vi "filter.debug.vi"(11 "filter.data in":T1 {"memory.command"."order.slot.value"."Quantity" format="%016x"; "memory.command"."order.slot.value"."OrderId" format="%016x"; "memory.command"."ticker.slot.value"."Symbol" format="%016x"; "Scratch"."OrderId" format="%016x"}) -> (3 "filter.data out":T1 {"memory.command"."order.slot.value"."Quantity" format="%016x"; "memory.command"."order.slot.value"."OrderId" format="%016x"; "memory.command"."ticker.slot.value"."Symbol" format="%016x"; "Scratch"."OrderId" format="%016x"})   [LabVIEW 2022 SP3]
uses:
  filter.data.ctl
  filter.states.ctl
  filter.debug.ctl
  filter.debug.slot.ctl
  filter.data.scratch.ctl
  common/orderbook.command.ctl
  common/orderbook.command.type.ctl
  filter.memory.command.ctl
  ticker.slot.ctl
  order.slot.ctl
  filter.getstate.ctl
  filter.getstate.slot.ctl
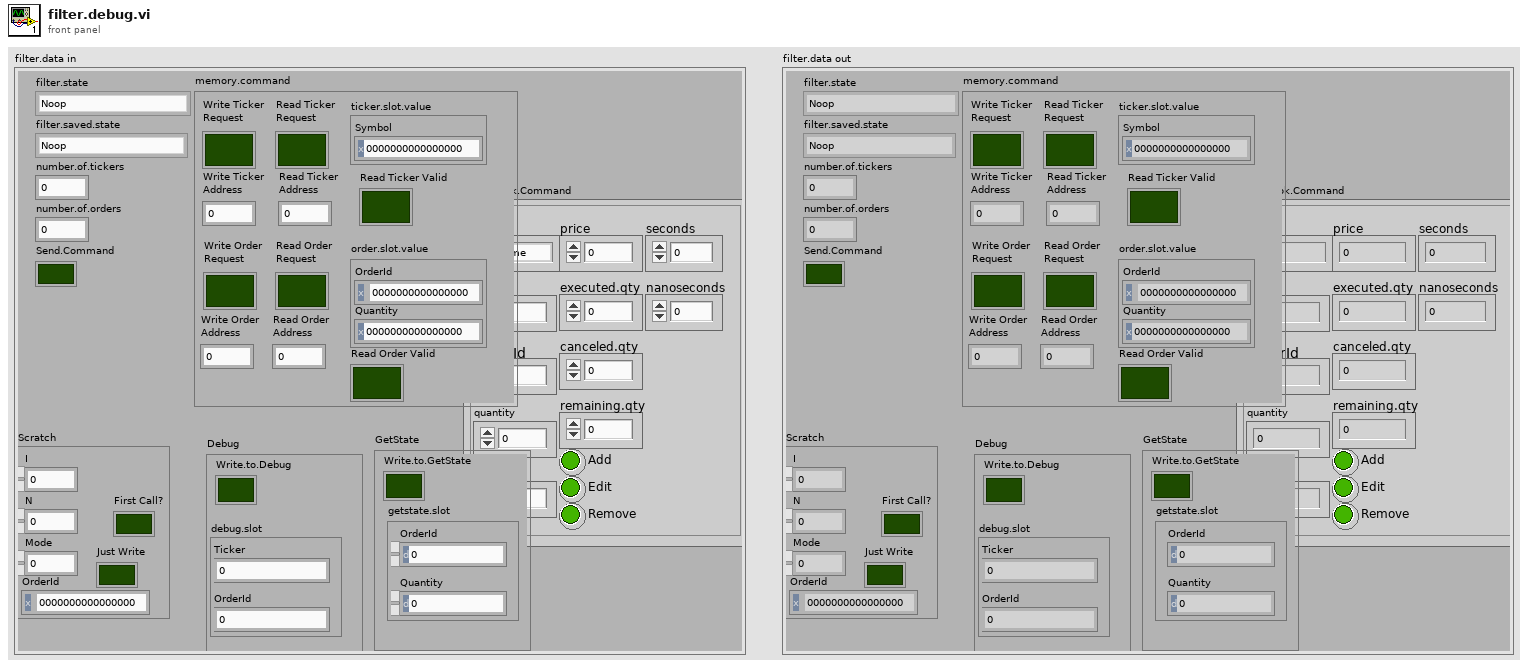
[diagram p1: front panel]
types:
  T1 = typedef "filter.data.ctl" = cluster{"filter.state":T2, "Debug":T3, "number.of.tickers":u32, "number.of.orders":u32, "filter.saved.state":T2, "Scratch":T5, "OrderBook.Command":T6, "Send.Command":bool, "memory.command":T8, "GetState":T11}
  T2 = typedef "filter.states.ctl" = enum16{"Noop", "Reset", "Debug", "Configuration", "Get.State", "Wait.for.Command", "Filter.Add", "Filter.Other", "Insert.Order", "Delete Order"}
  T3 = typedef "filter.debug.ctl" = cluster{"Write.to.Debug":bool, "debug.slot":T4}
  T4 = typedef "filter.debug.slot.ctl" = cluster{"Ticker":u64, "OrderId":u64}
  T5 = typedef "filter.data.scratch.ctl" = cluster{"I":u32, "N":u32, "Mode":u32, "OrderId":u64, "First Call?":bool, "Just Write":bool}
  T6 = typedef "orderbook.command.ctl" = cluster{"type":T7, "side":u8, "orderId ":u64, "quantity":u32, "symbol":u64, "price":u64, "executed.qty":u32, "canceled.qty":u32, "remaining.qty":u32, "seconds":u64, "nanoseconds":u64, "Add":bool, "Edit":bool, "Remove":bool}
  T7 = typedef "orderbook.command.type.ctl" = enum8{"Time", "AddOrder", "OrderExecuted", "OrderExecutedAtPrice", "ReduceSize", "ModifyOrder", "DeleteOrder", "Get.Everything", "Get.All.Orders", "Get.Top"}
  T8 = typedef "filter.memory.command.ctl" = cluster{"ticker.slot.value":T9, "order.slot.value":T10, "Write Ticker\nAddress":u32, "Write Ticker\nRequest":bool, "Read Ticker\nRequest":bool, "Read Ticker\nAddress":u32, "Read Ticker Valid":bool, "Write Order\nAddress":u32, "Write Order\nRequest":bool, "Read Order\nRequest":bool, "Read Order\nAddress":u32, "Read Order Valid":bool}
  T9 = typedef "ticker.slot.ctl" = cluster{"Symbol":u64}
  T10 = typedef "order.slot.ctl" = cluster{"OrderId":u64, "Quantity":u64}
  T11 = typedef "filter.getstate.ctl" = cluster{"Write.to.GetState":bool, "getstate.slot":T12}
  T12 = typedef "filter.getstate.slot.ctl" = cluster{"OrderId":u64, "Quantity":u64}
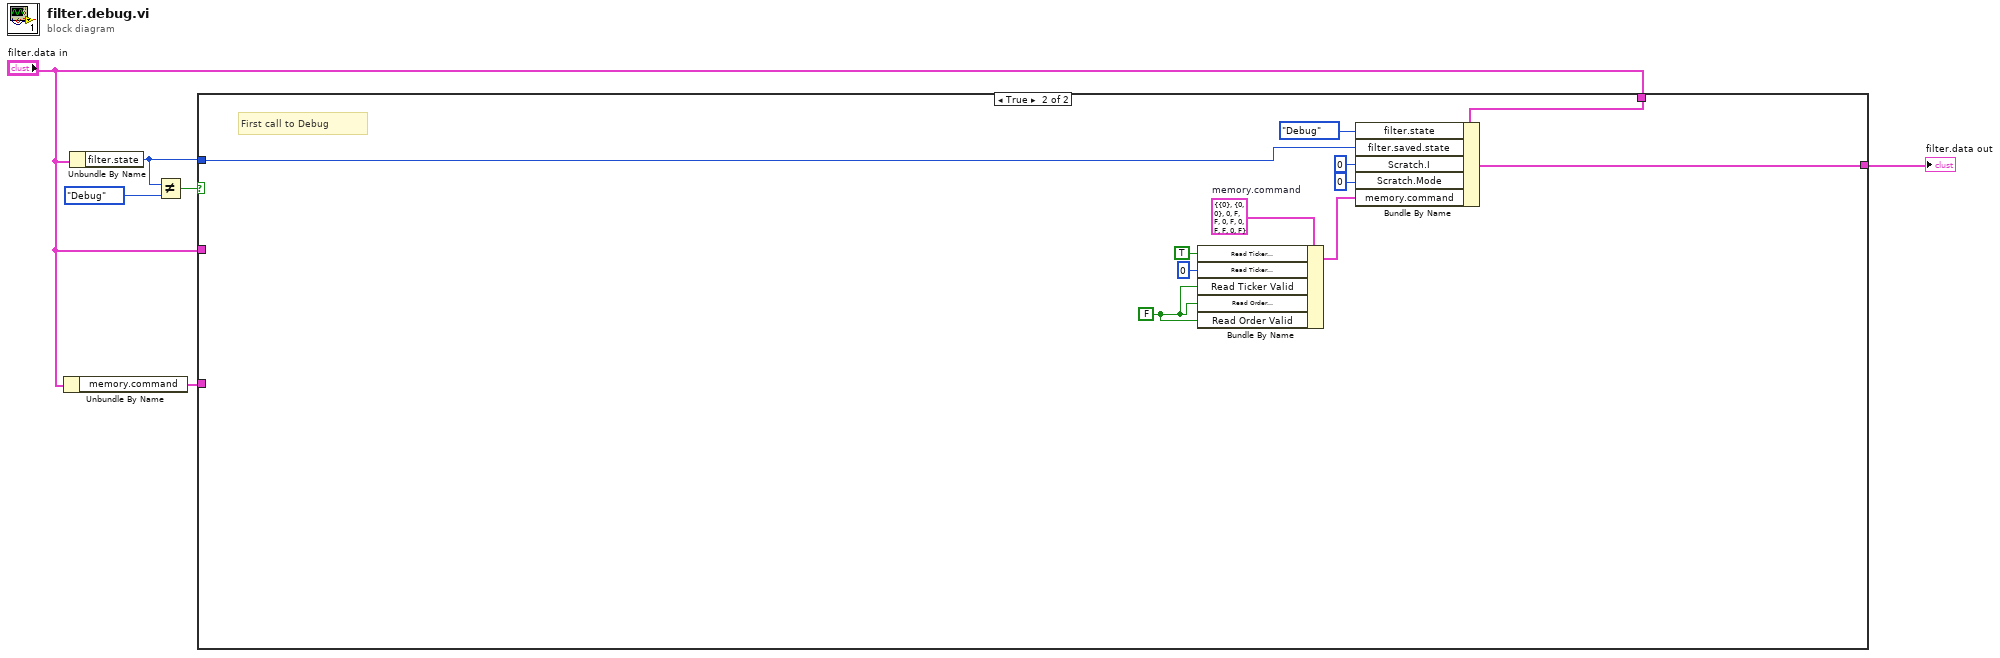
[diagram p0: block diagram]
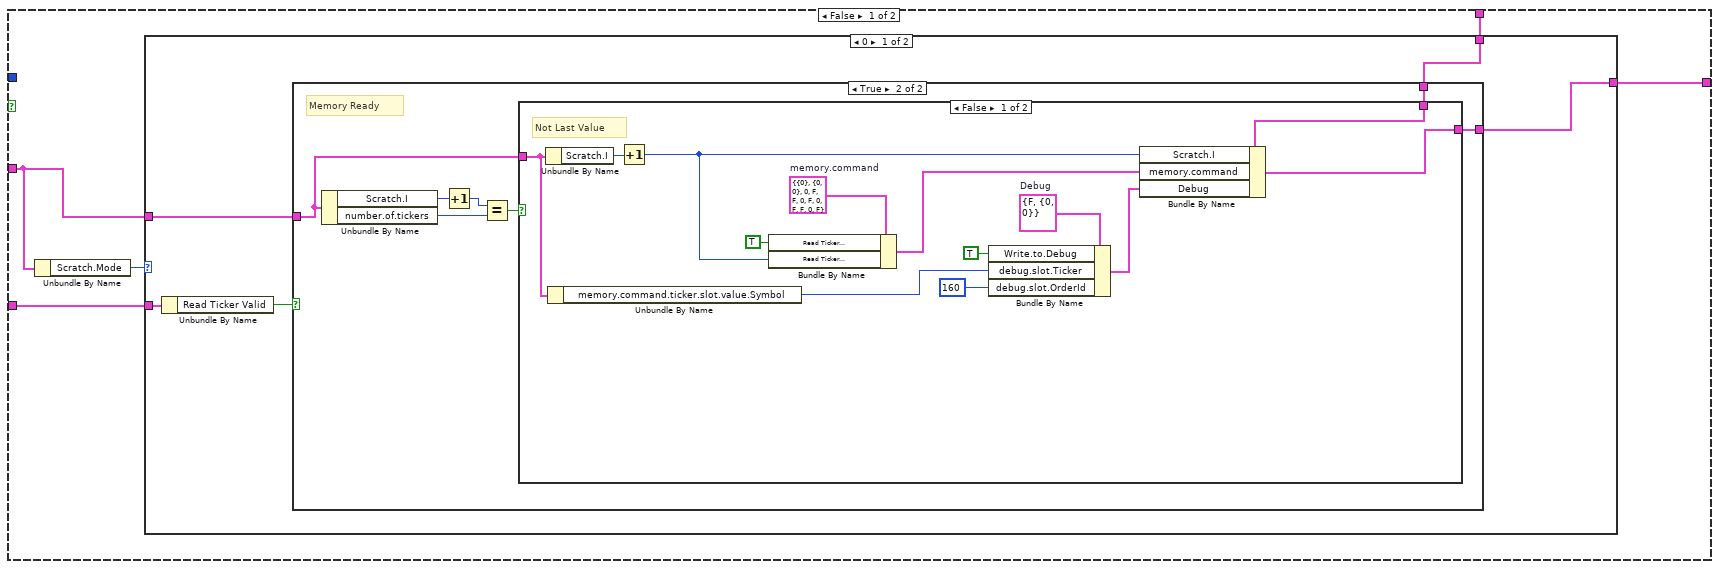
[diagram p2: hidden frame]
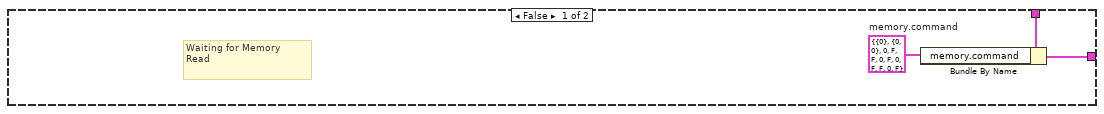
[diagram p3: hidden frame]
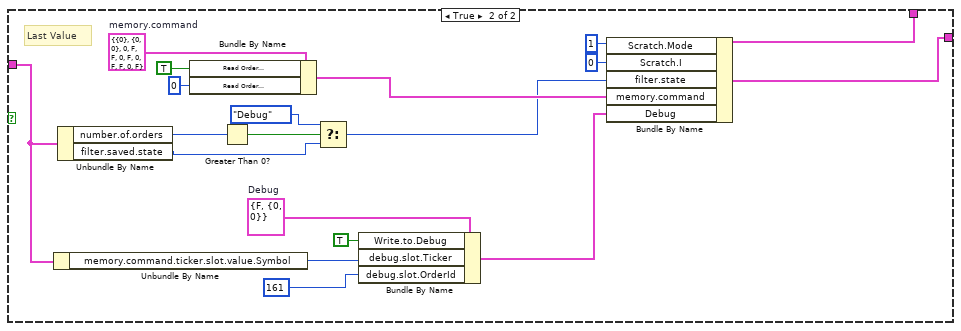
[diagram p4: hidden frame]
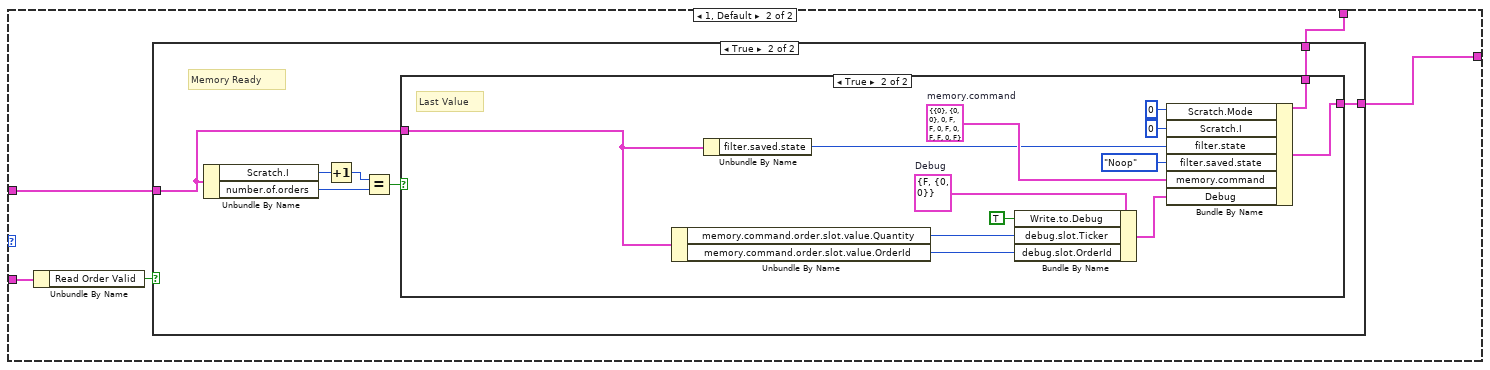
[diagram p5: hidden frame]
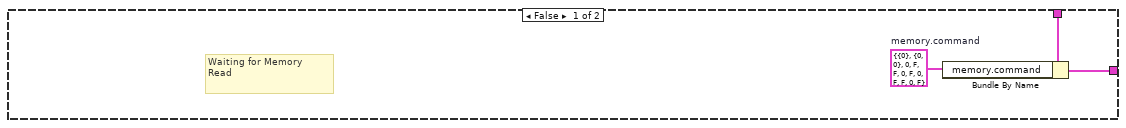
[diagram p6: hidden frame]
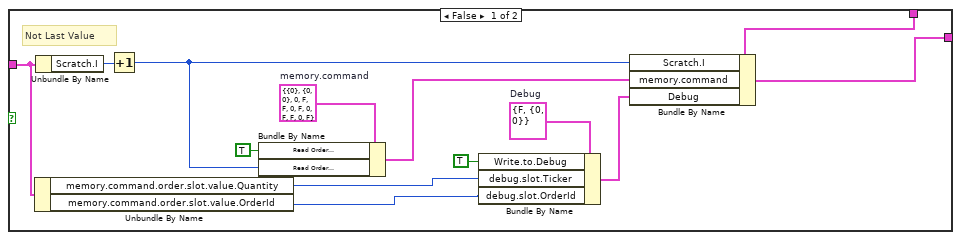
[diagram p7: hidden frame]
diagram:
  n1 = Unbundle By Name("filter.data in") -> ("memory.command"=w5:T8)
  n2 = Unbundle By Name("filter.data in") -> ("filter.state"=w3:T2)
  n3 = Not Equal?(x=w3, y=filter.states."Debug" ("filter.state")) -> (x != y?=w2:bool)
  n4 = case shown="True" w2 {
    tunnel: "filter.data in" -> [w10 w110]
    tunnel: [w11 w109] -> w1
    tunnel: w3 -> [_ w107]
    tunnel: "filter.data in" -> [w8 _]
    tunnel: w5 -> [w9 _]
    frame False {
      n5 = Unbundle By Name(w8) -> ("Scratch.Mode"=w7:u32)
      n6 = case shown="0" w7 {
        tunnel: [w16 w63] -> w11
        tunnel: w10 -> [w15 w62]
        tunnel: w9 -> [w13 w60]
        tunnel: w8 -> [w12 w59]
        frame 0 {
          n7 = Unbundle By Name(w13) -> ("Read Ticker Valid"=w14:bool)
          n8 = case shown="True" w14 {
            tunnel: [w17 w20] -> w16
            tunnel: w15 -> [w19 w21]
            tunnel: w12 -> [_ w22]
            frame False {
              w18 = T8 {"ticker.slot.value"={"Symbol"=0}, "order.slot.value"={"OrderId"=0, "Quantity"=0}, "Write Ticker\nAddress"=0, "Write Ticker\nRequest"=FALSE, "Read Ticker\nRequest"=FALSE, "Read Ticker\nAddress"=0, "Read Ticker Valid"=FALSE, "Write Order\nAddress"=0, "Write Order\nRequest"=FALSE, "Read Order\nRequest"=FALSE, "Read Order\nAddress"=0, "Read Order Valid"=FALSE}  # memory.command
              # "Waiting for Memory\nRead"
              n9 = Bundle By Name(cluster=w19, "memory.command"=w18) -> (w17:T1)
            }
            frame True {
              # "Memory Ready"
              n10 = Unbundle By Name(w22) -> ("Scratch.I"=w26:u32, "number.of.tickers"=w24:u32)
              n11 = Increment(x=w26) -> (x+1=w25:u32)
              n12 = Equal?(x=w25, y=w24) -> (x = y?=w23:bool)
              n13 = case shown="False" w23 {
                tunnel: w22 -> [w32 w45]
                tunnel: w21 -> [w28 w58]
                tunnel: [w39 w57] -> w20
                frame False {
                  w35 = T3 {"Write.to.Debug"=FALSE, "debug.slot"={"Ticker"=0, "OrderId"=0}}  # Debug
                  w38 = T8 {"ticker.slot.value"={"Symbol"=0}, "order.slot.value"={"OrderId"=0, "Quantity"=0}, "Write Ticker\nAddress"=0, "Write Ticker\nRequest"=FALSE, "Read Ticker\nRequest"=FALSE, "Read Ticker\nAddress"=0, "Read Ticker Valid"=FALSE, "Write Order\nAddress"=0, "Write Order\nRequest"=FALSE, "Read Order\nRequest"=FALSE, "Read Order\nAddress"=0, "Read Order Valid"=FALSE}  # memory.command
                  # "Not Last Value"
                  n14 = Unbundle By Name(w32) -> ("Scratch.I"=w36:u32)
                  n15 = Unbundle By Name(w32) -> ("memory.command.ticker.slot.value.Symbol"=w31:u64)
                  n16 = Increment(x=w36) -> (x+1=w29:u32)
                  n17 = Bundle By Name(cluster=w38, "Read Ticker\nRequest"=TRUE ("Read.Request"), "Read Ticker\nAddress"=w29) -> (w37:T8)
                  n18 = Bundle By Name(cluster=w35, "Write.to.Debug"=TRUE, "debug.slot.Ticker"=w31, "debug.slot.OrderId"=u64 160) -> (w34:T3)
                  n19 = Bundle By Name(cluster=w28, "Scratch.I"=w29, "memory.command"=w37, "Debug"=w34) -> (w39:T1)
                }
                frame True {
                  w56 = T3 {"Write.to.Debug"=FALSE, "debug.slot"={"Ticker"=0, "OrderId"=0}}  # Debug
                  w49 = T8 {"ticker.slot.value"={"Symbol"=0}, "order.slot.value"={"OrderId"=0, "Quantity"=0}, "Write Ticker\nAddress"=0, "Write Ticker\nRequest"=FALSE, "Read Ticker\nRequest"=FALSE, "Read Ticker\nAddress"=0, "Read Ticker Valid"=FALSE, "Write Order\nAddress"=0, "Write Order\nRequest"=FALSE, "Read Order\nRequest"=FALSE, "Read Order\nAddress"=0, "Read Order Valid"=FALSE}  # memory.command
                  # "Last Value"
                  n20 = Unbundle By Name(w45) -> ("memory.command.ticker.slot.value.Symbol"=w53:u64)
                  n21 = Unbundle By Name(w45) -> ("number.of.orders"=w44:u32, "filter.saved.state"=w40:T2)
                  n22 = Bundle By Name(cluster=w49, "Read Order\nRequest"=TRUE ("Read Order\nRequest"), "Read Order\nAddress"=u32 0 ("Read Order\nAddress")) -> (w48:T8)
                  n23 = Greater Than 0?(x=w44) -> (x > 0?=w43:bool)
                  n24 = Select(t=filter.states."Debug" ("filter.state"), s=w43, f=w40) -> (s? t:f=w41:T2)
                  n25 = Bundle By Name(cluster=w56, "Write.to.Debug"=TRUE, "debug.slot.Ticker"=w53, "debug.slot.OrderId"=u64 161) -> (w55:T3)
                  n26 = Bundle By Name(cluster=w58, "Scratch.Mode"=u32 1, "Scratch.I"=u32 0, "filter.state"=w41, "memory.command"=w48, "Debug"=w55) -> (w57:T1)
                }
              }
            }
          }
        }
        frame 1, Default {
          n27 = Unbundle By Name(w60) -> ("Read Order Valid"=w61:bool)
          n28 = case shown="True" w61 {
            tunnel: [w64 w67] -> w63
            tunnel: w62 -> [w66 w68]
            tunnel: w59 -> [_ w69]
            frame False {
              w65 = T8 {"ticker.slot.value"={"Symbol"=0}, "order.slot.value"={"OrderId"=0, "Quantity"=0}, "Write Ticker\nAddress"=0, "Write Ticker\nRequest"=FALSE, "Read Ticker\nRequest"=FALSE, "Read Ticker\nAddress"=0, "Read Ticker Valid"=FALSE, "Write Order\nAddress"=0, "Write Order\nRequest"=FALSE, "Read Order\nRequest"=FALSE, "Read Order\nAddress"=0, "Read Order Valid"=FALSE}  # memory.command
              # "Waiting for Memory\nRead"
              n29 = Bundle By Name(cluster=w66, "memory.command"=w65) -> (w64:T1)
            }
            frame True {
              # "Memory Ready"
              n30 = Unbundle By Name(w69) -> ("Scratch.I"=w73:u32, "number.of.orders"=w71:u32)
              n31 = Increment(x=w73) -> (x+1=w72:u32)
              n32 = Equal?(x=w72, y=w71) -> (x = y?=w70:bool)
              n33 = case shown="True" w70 {
                tunnel: w69 -> [w79 w94]
                tunnel: w68 -> [w77 w99]
                tunnel: [w86 w98] -> w67
                frame False {
                  w82 = T3 {"Write.to.Debug"=FALSE, "debug.slot"={"Ticker"=0, "OrderId"=0}}  # Debug
                  w85 = T8 {"ticker.slot.value"={"Symbol"=0}, "order.slot.value"={"OrderId"=0, "Quantity"=0}, "Write Ticker\nAddress"=0, "Write Ticker\nRequest"=FALSE, "Read Ticker\nRequest"=FALSE, "Read Ticker\nAddress"=0, "Read Ticker Valid"=FALSE, "Write Order\nAddress"=0, "Write Order\nRequest"=FALSE, "Read Order\nRequest"=FALSE, "Read Order\nAddress"=0, "Read Order Valid"=FALSE}  # memory.command
                  # "Not Last Value"
                  n34 = Unbundle By Name(w79) -> ("memory.command.order.slot.value.Quantity"=w74:u64, "memory.command.order.slot.value.OrderId"=w75:u64)
                  n35 = Unbundle By Name(w79) -> ("Scratch.I"=w83:u32)
                  n36 = Increment(x=w83) -> (x+1=w76:u32)
                  n37 = Bundle By Name(cluster=w85, "Read Order\nRequest"=TRUE ("Read.Request"), "Read Order\nAddress"=w76) -> (w84:T8)
                  n38 = Bundle By Name(cluster=w82, "Write.to.Debug"=TRUE, "debug.slot.Ticker"=w74, "debug.slot.OrderId"=w75) -> (w81:T3)
                  n39 = Bundle By Name(cluster=w77, "Scratch.I"=w76, "memory.command"=w84, "Debug"=w81) -> (w86:T1)
                }
                frame True {
                  w97 = T3 {"Write.to.Debug"=FALSE, "debug.slot"={"Ticker"=0, "OrderId"=0}}  # Debug
                  w93 = T8 {"ticker.slot.value"={"Symbol"=0}, "order.slot.value"={"OrderId"=0, "Quantity"=0}, "Write Ticker\nAddress"=0, "Write Ticker\nRequest"=FALSE, "Read Ticker\nRequest"=FALSE, "Read Ticker\nAddress"=0, "Read Ticker Valid"=FALSE, "Write Order\nAddress"=0, "Write Order\nRequest"=FALSE, "Read Order\nRequest"=FALSE, "Read Order\nAddress"=0, "Read Order Valid"=FALSE}  # memory.command
                  # "Last Value"
                  n40 = Unbundle By Name(w94) -> ("memory.command.order.slot.value.Quantity"=w88:u64, "memory.command.order.slot.value.OrderId"=w87:u64)
                  n41 = Unbundle By Name(w94) -> ("filter.saved.state"=w92:T2)
                  n42 = Bundle By Name(cluster=w97, "Write.to.Debug"=TRUE, "debug.slot.Ticker"=w88, "debug.slot.OrderId"=w87) -> (w96:T3)
                  n43 = Bundle By Name(cluster=w99, "Scratch.Mode"=u32 0, "Scratch.I"=u32 0, "filter.state"=w92, "filter.saved.state"=filter.states."Noop", "memory.command"=w93, "Debug"=w96) -> (w98:T1)
                }
              }
            }
          }
        }
      }
    }
    frame True {
      w101 = FALSE ("Read Ticker Valid")
      w103 = T8 {"ticker.slot.value"={"Symbol"=0}, "order.slot.value"={"OrderId"=0, "Quantity"=0}, "Write Ticker\nAddress"=0, "Write Ticker\nRequest"=FALSE, "Read Ticker\nRequest"=FALSE, "Read Ticker\nAddress"=0, "Read Ticker Valid"=FALSE, "Write Order\nAddress"=0, "Write Order\nRequest"=FALSE, "Read Order\nRequest"=FALSE, "Read Order\nAddress"=0, "Read Order Valid"=FALSE}  # memory.command
      # "First call to Debug"
      n44 = Bundle By Name(cluster=w103, "Read Ticker\nRequest"=TRUE ("Read Ticker\nRequest"), "Read Ticker\nAddress"=u32 0 ("Read Ticker\nAddress"), "Read Ticker Valid"=w101, "Read Order\nRequest"=w101, "Read Order Valid"=w101) -> (w104:T8)
      n45 = Bundle By Name(cluster=w110, "filter.state"=filter.states."Debug", "filter.saved.state"=w107, "Scratch.I"=u32 0, "Scratch.Mode"=u32 0, "memory.command"=w104) -> (w109:T1)
    }
  }
  "filter.data out" <- w1
